vi "SubVI_Write_Allan_Result_TDMS.vi"(0 "error in":errorcluster caption="错误输入（无错误）", 2 "TDMS保存路径":path, 3 "num_pairs":dbl[](array[numeric]), 4 "allan_variance":dbl[](array[numeric]), 5 "allan_deviation":dbl[](array[numeric]), 6 "tau_s":dbl[](array[numeric])) -> (1 "error out":errorcluster caption="错误输出")   [LabVIEW 2024]
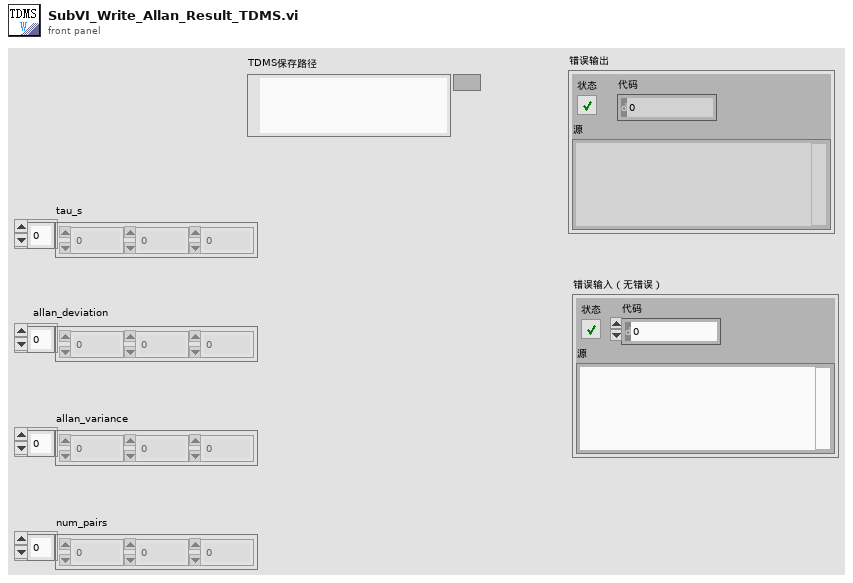
[diagram p1: front panel]
types:
  T1 = enum16{"open", "open or create", "create or replace", "create", "open (read-only)"}
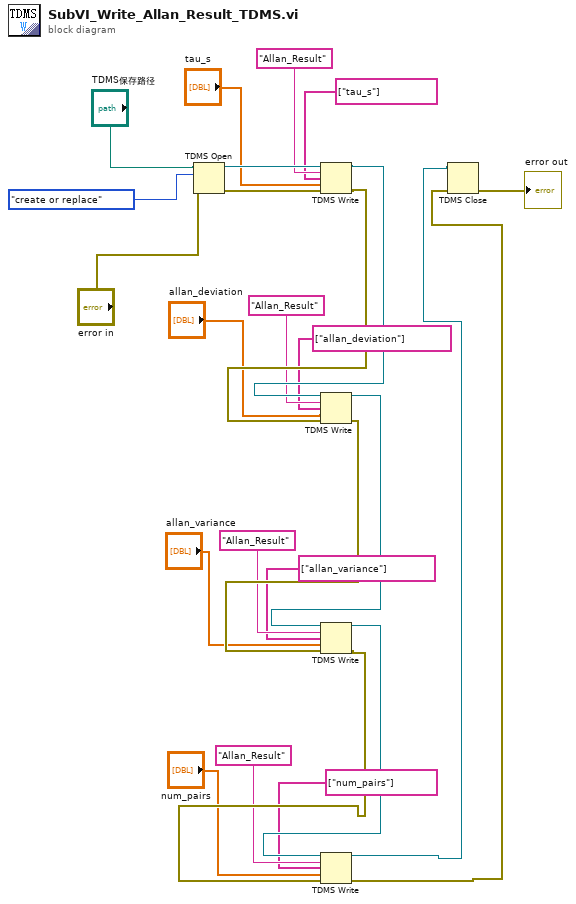
[diagram p0: block diagram]
diagram:
  n1 = TDMS Open(8:"error in", 10:T1."create or replace" ("操作(0:open)"), 11:"TDMS保存路径") -> (0:w22:errorcluster, 3:w23:refnum<k34>)  [unwired: 4 in]
  n2 = TDMS Write(0:w23, 5:"Allan_Result" ("组名称输入（无标题）"), 7:string[] ["tau_s"] ("通道名输入（无标题）"), 9:"tau_s", 11:w22) -> (4:w18:refnum<k34>, 15:w17:errorcluster)  [unwired: 1 in, 2 out]
  n3 = TDMS Write(0:w18, 5:"Allan_Result" ("组名称输入（无标题）"), 7:string[] ["allan_deviation"] ("通道名输入（无标题）"), 9:"allan_deviation", 11:w17) -> (4:w14:refnum<k34>, 15:w11:errorcluster)  [unwired: 1 in, 2 out]
  n4 = TDMS Write(0:w14, 5:"Allan_Result" ("组名称输入（无标题）"), 7:string[] ["allan_variance"] ("通道名输入（无标题）"), 9:"allan_variance", 11:w11) -> (4:w13:refnum<k34>, 15:w10:errorcluster)  [unwired: 1 in, 2 out]
  n5 = TDMS Write(0:w13, 5:"Allan_Result" ("组名称输入（无标题）"), 7:string[] ["num_pairs"] ("通道名输入（无标题）"), 9:"num_pairs", 11:w10) -> (4:w8:refnum<k34>, 15:w9:errorcluster)  [unwired: 1 in, 2 out]
  n6 = TDMS Close(8:w9, 11:w8) -> (0:→"error out":errorcluster)  [unwired: 1 out]
